vi "Write DC.vi"(8 "error in (no error)":errorcluster, 10 "DC":dbl, 11 "Change Blue Laser DC MSG in":refnum<class "Change Red DC MSG.lvclass">) -> (0 "error out":errorcluster, 3 "Change Blue Laser DC MSG out":refnum<class "Change Red DC MSG.lvclass">)   [LabVIEW 2014, in "eCRDS Library.lvlib" / "Change Red DC MSG.lvclass"]
uses:
  Change Red DC MSG.lvclass
  Change Red DC MSG.lvclass/Change Red DC MSG.ctl
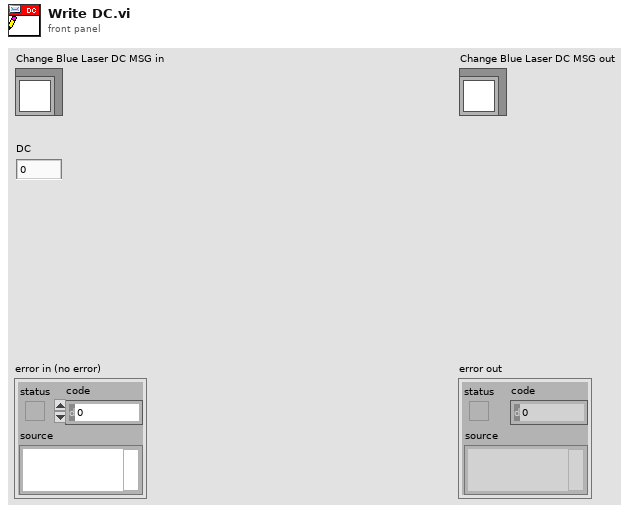
[diagram p1: front panel]
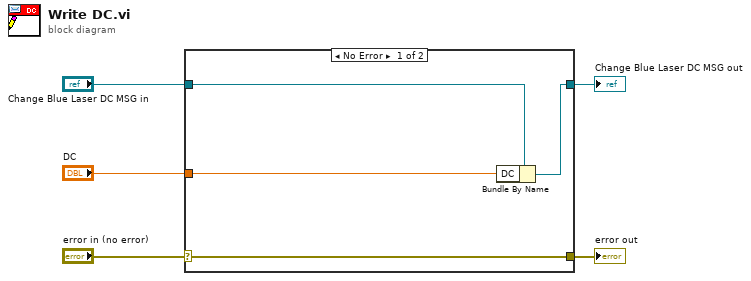
[diagram p0: block diagram]
diagram:
  n1 = case shown="No Error" "error in (no error)" {
    selector: "error in (no error)" -> [w9 w10]
    tunnel: [w9 w10] -> w4
    tunnel: [w7 w11] -> w2
    tunnel: "Change Blue Laser DC MSG in" -> [w8 w11]
    tunnel: "DC" -> [w6 _]
    frame No Error {
      n2 = Bundle By Name(cluster=w8, "DC"=w6) -> (w7:refnum<class "Change Red DC MSG.lvclass">)
    }
    frame Error {
    }
  }
  "error out" <- w4
  "Change Blue Laser DC MSG out" <- w2
